vi "习题7.2.vi"() -> ()   [LabVIEW 2017]
panel:
  out "波形图":cluster{dbl[]}[](graph)
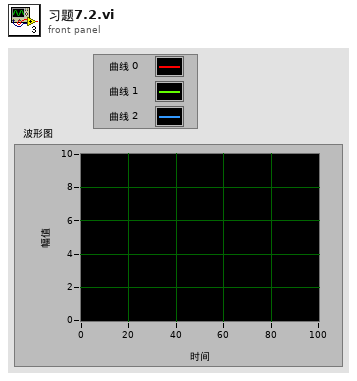
[diagram p1: front panel]
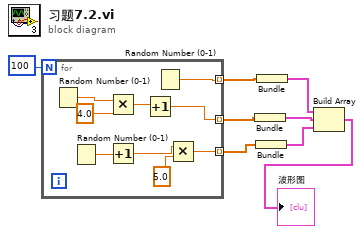
[diagram p0: block diagram]
diagram:
  n1 = for {
    N: 100 -> [_]
    tunnel: [w9] -> w7 mode=indexing
    tunnel: [w14] -> w6 mode=indexing
    tunnel: [w11] -> w5 mode=indexing
    n2 = Random Number (0-1)() -> (number: 0 to 1=w16:dbl)
    n3 = Random Number (0-1)() -> (number: 0 to 1=w13:dbl)
    n4 = Multiply(x=w16, y=4.0) -> (x*y=w17:dbl)
    n5 = Increment(x=w13) -> (x+1=w10:dbl)
    n6 = Increment(x=w17) -> (x+1=w14:dbl)
    n7 = Random Number (0-1)() -> (number: 0 to 1=w9:dbl)
    n8 = Multiply(x=w10, y=5.0) -> (x*y=w11:dbl)
  }
  n9 = Bundle(w6) -> (w1:cluster{dbl[]})  [unwired: 1 in]
  n10 = Bundle(w5) -> (w3:cluster{dbl[]})  [unwired: 1 in]
  n11 = Bundle(w7) -> (w4:cluster{dbl[]})  [unwired: 1 in]
  n12 = Build Array(w4, w1, w3) -> (→"波形图":cluster{dbl[]}[])
